vi "uActor_Enable AutoACK.vi"(8 "error in (no error)":errorcluster, 11 "uActor in":refnum<class "uActor.lvclass">) -> (0 "error out":errorcluster, 3 "uActor out":refnum<class "uActor.lvclass">)   [LabVIEW 2023, in "uLib.lvlib" / "uActor.lvclass"]
doc: "Call this method to enable an actor to send auto ack messages or auto reply meesages as it processes the incoming commands in the EXEC method.\n\nThis is relevant for most actors OR for observers that take ownership of processing specific message, ideally distinguished by a predetermined prefix. This excludes observers who monitors all topics but should not actively send out an acknowledgement or a reply."
uses:
  uActor.lvclass
  uActor.lvclass/uActor.ctl
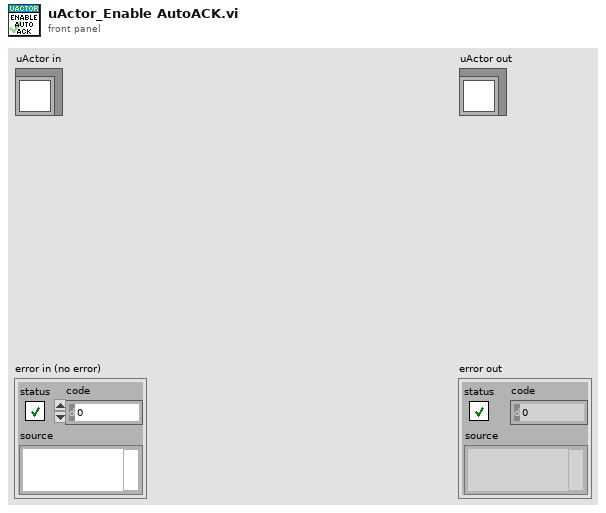
[diagram p1: front panel]
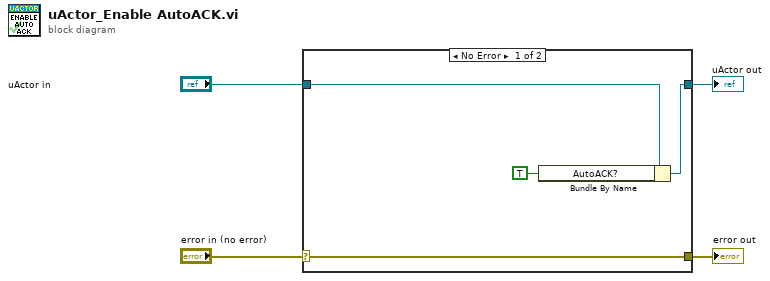
[diagram p0: block diagram]
diagram:
  n1 = case shown="No Error" "error in (no error)" {
    selector: "error in (no error)" -> [w8 w9]
    tunnel: [w8 w9] -> w3
    tunnel: [w6 w10] -> w1
    tunnel: "uActor in" -> [w7 w10]
    frame No Error {
      n2 = Bundle By Name(cluster=w7, "AutoACK?"=TRUE ("RnT config.AutoACK?")) -> (w6:refnum<class "uActor.lvclass">)
    }
    frame Error {
    }
  }
  "error out" <- w3
  "uActor out" <- w1
